vi "N-Memory write from DMA - Target.vi"(9 "n":u32=1) -> ()   [LabVIEW 2014]
uses:
  <vilib>/rvi/Emulation/niFpgaGetClockAttributes.vi
  <vilib>/rvi/Emulation/niFpgaSctlEmulationGetInTimedLoop.vi
  <vilib>/rvi/Emulation/niFpgaEmulationReportErrorSimple.vi
  <vilib>/rvi/interface/RandomDataEmulation/niFpgaRandomDataHandleErrors.vi
  <vilib>/rvi/Memory/Memory_Emulation/nirvimemoryFastEmulation.vi
  <vilib>/rvi/Memory/Memory_Emulation/nirvimemoryEmulation.vi
  <vilib>/rvi/Emulation/niFpgaEmulationIsFPGAContextNoSignature.vi
  <vilib>/rvi/DataTransferAndStorage/Container/Common/niFpgaContainerGetUniqueNameForEmu.vi
  <vilib>/rvi/Emulation/niFpgaProcessEmulError.vi
  <vilib>/rvi/errors/nirviReportUnexpectedCaseInternalError (U32).vi
  <vilib>/rvi/Emulation/niFpgaCriticalErrorInLSC.vi
  <vilib>/rvi/DataTransferAndStorage/Container/XNode/niFpgaContainer.xnode
  <vilib>/rvi/interface/RandomDataEmulation/nirviRandomDataFpgaReadWriteTemplate.vi
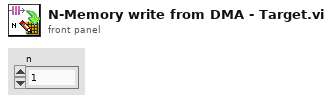
[diagram p1: front panel]
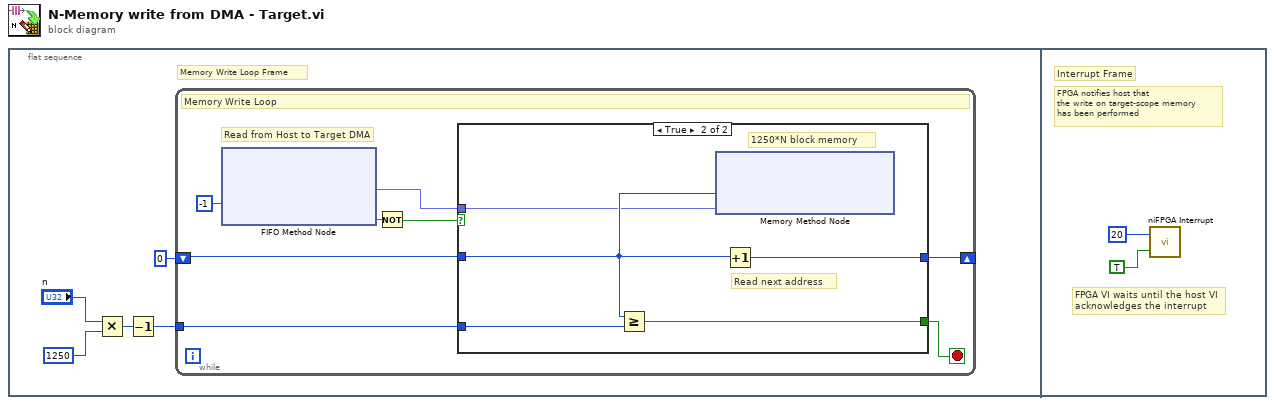
[diagram p0: block diagram]
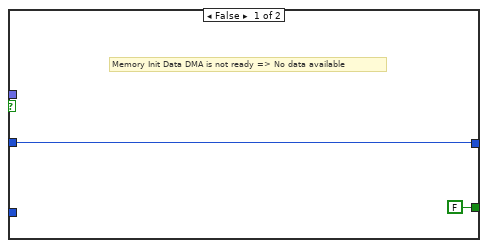
[diagram p2: hidden frame]
diagram:
  n1 = flat-sequence {
    frame #0 {
      # "Memory Write Loop Frame"
      n2 = Multiply(x="n", y=u32 1250) -> (x*y=w2:u32)
      n3 = Decrement(x=w2) -> (x-1=w1:u32)
      n4 = while {
        shift-right: [w11] -> _
        shift-left: u32 0 -> [w12]
        tunnel: w1 -> [w6]
        stop <- w13 stop-if-true
        # "Read from Host to Target DMA"
        # "Memory Write Loop"
        n5 = xnode ("FIFO Method Node")("Timeout"=-1) -> ("Element"=w7:fxp<+/-,12,12>, "Timed Out?"=w9:bool)  [unwired: 1 in, 1 out]
        n6 = Not(x=w9) -> (.not. x?=w8:bool)
        n7 = case shown="True" w8 {
          tunnel: [FALSE w20] -> w13
          tunnel: w12 -> [w14 w19]
          tunnel: [w14 w18] -> w11
          tunnel: w7 -> [_ w17]
          tunnel: w6 -> [_ w16]
          frame False {
            # "Memory Init Data DMA is not ready => No data available"
          }
          frame True {
            # "Read next address"
            # "1250*N block memory"
            n8 = Greater Or Equal?(x=w19, y=w16) -> (x >= y?=w20:bool)
            n9 = xnode ("Memory Method Node")("Address"=w19, "Data"=w17) -> ()  [unwired: 1 in, 1 out]
            n10 = Increment(x=w19) -> (x+1=w18:u32)
          }
        }
      }
    }
    frame #1 {
      # "FPGA VI waits until the host VI \nacknowledges the interrupt"
      # "FPGA notifies host that\nthe write on target-scope memory\nhas been performed"
      # "Interrupt Frame"
      n11 = call <vilib>:"niFPGA Interrupt.vi"("Wait Until Cleared (F)"=TRUE, "IRQ Number (0)"=u8 20) -> ()  [unwired: 1 in]
    }
  }
